vi "BRAM_ReadBlockMask.vi"(2 "Address":i16) -> (16 "PixelData":bool[](array[boolean]))   [LabVIEW 2018]
uses:
  <vilib>/rvi/Memory/Memory_Emulation/nirvimemoryFastEmulation.vi
  <vilib>/rvi/Memory/Memory_Emulation/nirvimemoryEmulation.vi
  <vilib>/rvi/Emulation/niFpgaEmulationIsFPGAContextNoSignature.vi
  <vilib>/rvi/DataTransferAndStorage/Container/Common/niFpgaContainerGetUniqueNameForEmu.vi
  <vilib>/rvi/Emulation/niFpgaProcessEmulError.vi
  <vilib>/rvi/Emulation/niFpgaSctlEmulationGetInTimedLoop.vi
  <vilib>/rvi/errors/nirviReportUnexpectedCaseInternalError (U32).vi
  <vilib>/rvi/DataTransferAndStorage/Container/XNode/niFpgaContainer.xnode
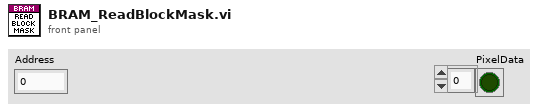
[diagram p1: front panel]
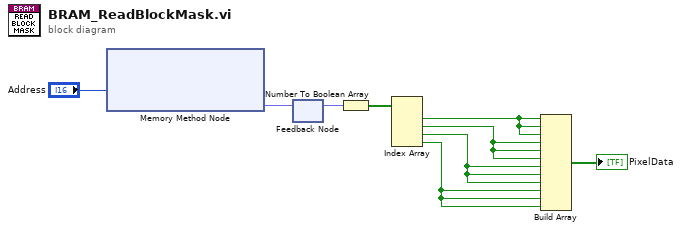
[diagram p0: block diagram]
diagram:
  n1 = xnode ("Memory Method Node")("Address A"="Address") -> ("Data A"=w1:fxp<+,4,4>)  [unwired: 1 in, 1 out]
  n2 = feedback #1() -> (w8:fxp<+,4,4>)  [unwired: 1 in]
  n3 = feedback-in #1(w1) -> ()
  n4 = Number To Boolean Array(number=w8) -> (Boolean array=w3:bool[])
  n5 = Index Array(array=w3) -> (element #1=w4:bool, element #2=w7:bool, element #3=w6:bool, element #4=w5:bool)  [unwired: 4 in]
  n6 = Build Array(w4, w4, w4, w7, w7, w7, w6, w6, w6, w5, w5, w5) -> (→"PixelData":bool[])
